vi "WriteScript.vi"() -> ()   [LabVIEW 2015]
panel:
  in  "text file":refnum<file>
  in  "Script Name":string
  out "status":string
  in  "Add to Script Button":bool
  in  "Location of Script File":path
  in  "cluster":T1={"Path to Configuration File"=path "", "SI camera info"={"Exp time"=0.0, "Number of Exp"=0.0, "Exp type tab"=enum."Object", "CCD ROI Mode"=10, "File name base"="", "Camera Color"="Red", "Notes"="", "Observer Name"="", "object name"="", "CCD Readout Speed"=5, "Hg(Ar)"=FALSE, "Cu"=FALSE, "Ne"=FALSE, "Ar"=FALSE, "Quartz"=FALSE, "Fe"=FALSE, "Bulb"=FALSE}} {"SI camera info"."CCD Readout Speed" items=["750 kHz, ATTN 0", "750 kHz, ATTN 2", "344 kHz, ATTN 0", "344 kHz, ATTN 3", "100 kHz, ATTN 2", "100 kHz, ATTN 3"]; "SI camera info"."CCD ROI Mode" items=["Imaging, 1x1  "=0, "Imaging, 2x2"=1, "Imaging, 3x3"=2, "Spectroscopic, 1x1"=3, "Spectroscopic, 2x2"=4, "Spectroscopic, 3x3"=5, "MOS, 1x1"=11, "MOS, 2x2"=12, "MOS, 3x3"=13, "Slicer"=6, "Spectroscopic, ZZ Ceti"=14, "Slit Imaging/Alignment"=7, "MOS Imaging/Alignment"=10, "Set user-defined ROI..."=8, "Custom Mode"=9]}
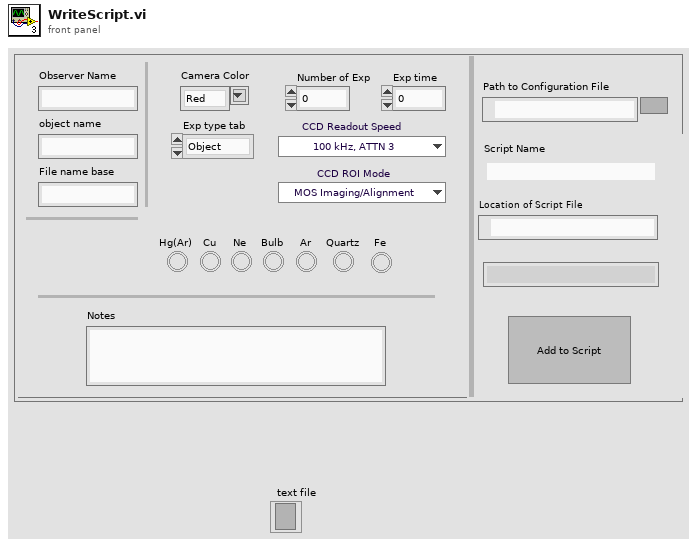
[diagram p1: front panel]
types:
  T1 = cluster{"Path to Configuration File":path, "SI camera info":cluster{"Exp time":dbl, "Number of Exp":dbl, "Exp type tab":enum16{"Object", "Flat", "Comp", "Dark", "Zero"}, "CCD ROI Mode":u16, "File name base":string, "Camera Color":string, "Notes":string, "Observer Name":string, "object name":string, "CCD Readout Speed":u8, "Hg(Ar)":bool, "Cu":bool, "Ne":bool, "Ar":bool, "Quartz":bool, "Fe":bool, "Bulb":bool}}
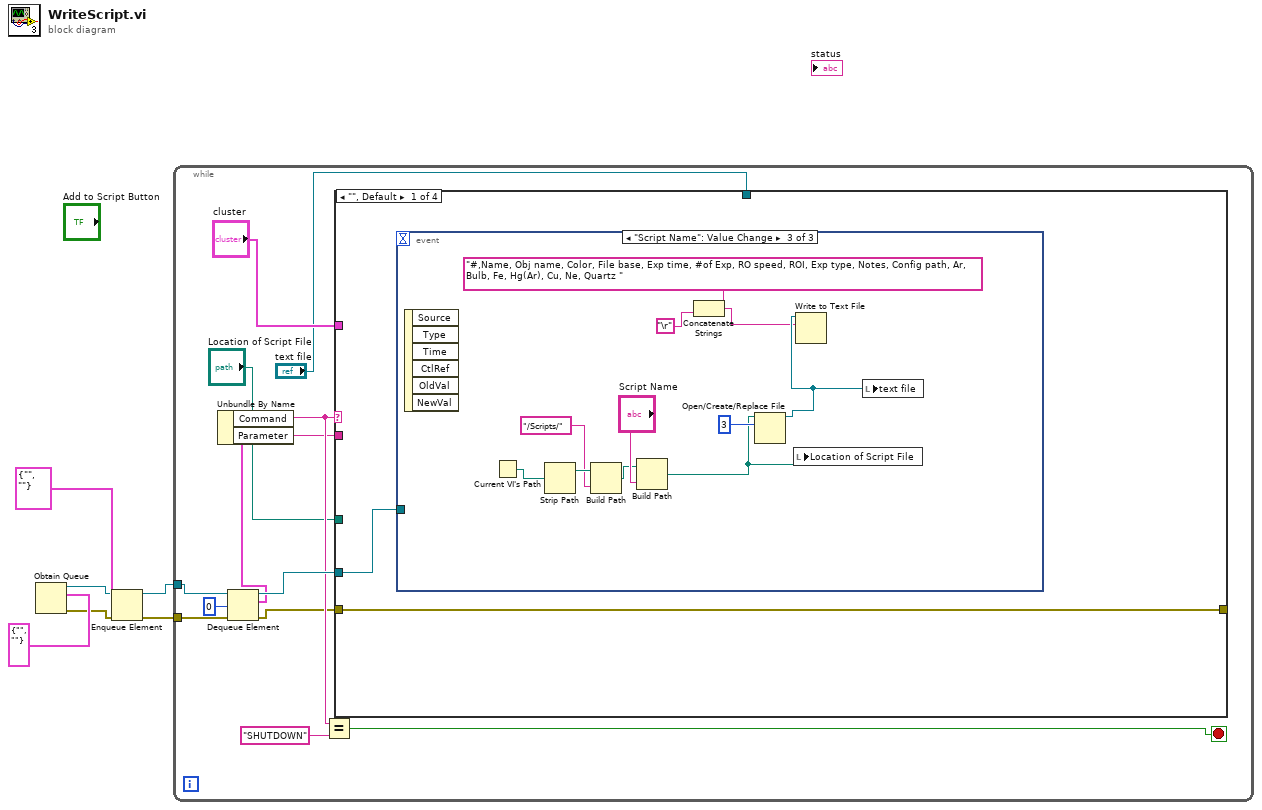
[diagram p0: block diagram]
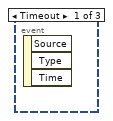
[diagram p2: hidden frame]
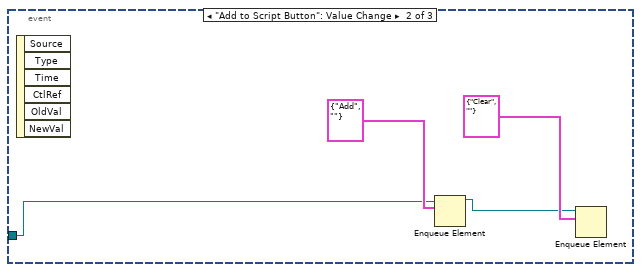
[diagram p3: hidden frame]
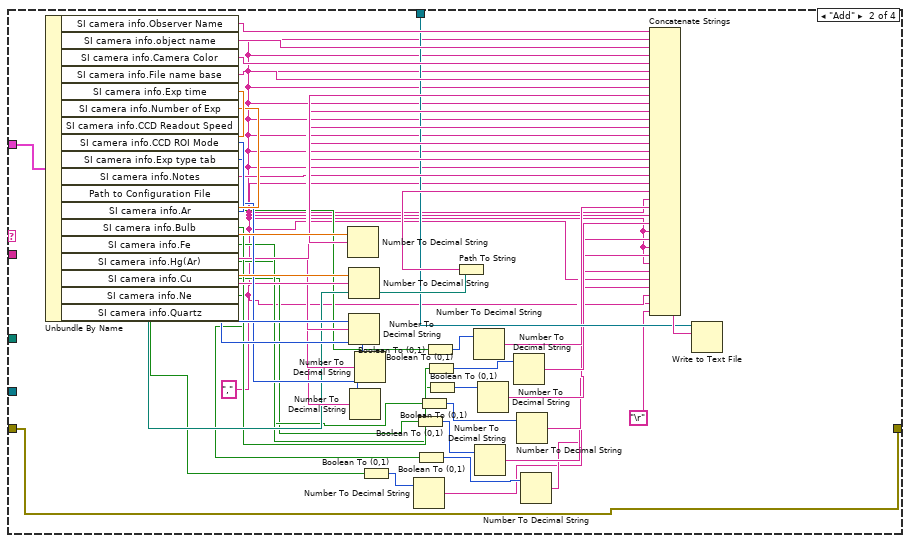
[diagram p4: hidden frame]
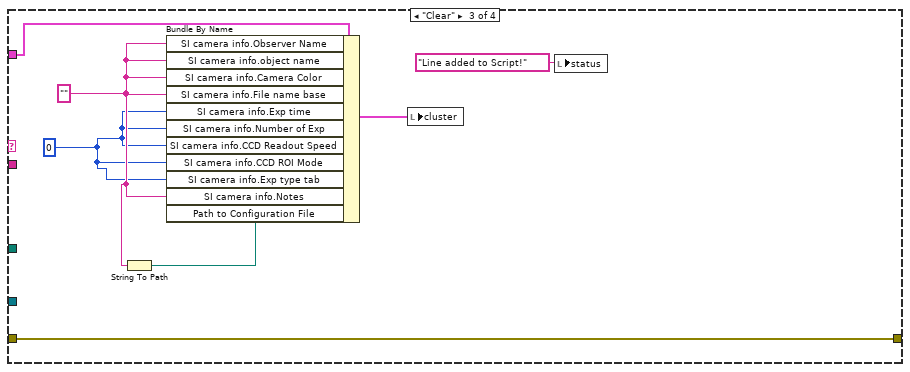
[diagram p5: hidden frame]
diagram:
  n1 = Obtain Queue(element data type=cluster{"\nCommand":string, "Parameter":string} {"\nCommand"="", "Parameter"=""}) -> (queue out=w4:refnum<queue>, error out=w2:errorcluster)  [unwired: 4 in, 1 out]
  n2 = Enqueue Element(queue=w4, element=cluster{string, string} {"", ""}, error in (no error)=w2) -> (queue out=w3:refnum<queue>, error out=w1:errorcluster)  [unwired: 1 in, 1 out]
  n3 = while {
    tunnel: w3 -> [w11]
    tunnel: w1 -> [w10]
    stop <- w15 stop-if-true
    n4 = Dequeue Element(queue=w11, timeout in ms (-1)=0, error in (no error)=w10) -> (queue out=w19:refnum<queue>, element=w18:cluster{"\nCommand":string, "Parameter":string}, error out=w9:errorcluster)  [unwired: 1 out]
    n5 = Unbundle By Name(w18) -> ("Command"=w16:string, "Parameter"=w14:string)
    n6 = Equal?(x=w16, y="SHUTDOWN") -> (x = y?=w15:bool)
    n7 = case shown="\"\", Default" w16 {
      tunnel: w19 -> [w21 _ _ _]
      tunnel: w14 -> [_ _ _ _]
      tunnel: "cluster" -> [_ w80 w87 _]
      tunnel: "Location of Script File" -> [_ _ _ _]
      tunnel: w9 -> [w20 w61 w83 w88]
      tunnel: [w20 w61 w83 w88] -> _
      tunnel: "text file" -> [_ w60 _ _]
      frame "", Default {
        n8 = event shown="[2] \"Script Name\": Value Change" {
          selector: _ -> [_ _ _]
          dyn-events: _ -> [_ _ _]
          timeout: _ -> [_ _ _]
          tunnel: w21 -> [_ w24 _]
          event Timeout {
            n9 = event-data() -> ()  [unwired: 1 in, 3 out]
          }
          event "Add to Script Button": Value Change {
            n10 = event-data() -> ()  [unwired: 1 in, 6 out]
            n11 = Enqueue Element(queue=w24, element=cluster{string, string} {"Add", ""}) -> (queue out=w22:refnum<queue>)  [unwired: 2 in, 2 out]
            n12 = Enqueue Element(queue=w22, element=cluster{string, string} {"Clear", ""}) -> ()  [unwired: 2 in, 3 out]
          }
          event "Script Name": Value Change {
            n13 = event-data() -> ()  [unwired: 1 in, 6 out]
            n14 = Current VI's Path() -> (path=w35:path)
            n15 = Strip Path(path=w35) -> (stripped path=w28:path)  [unwired: 1 out]
            n16 = Build Path(base path=w28, name or relative path="/Scripts/") -> (appended path=w27:path)
            n17 = Build Path(base path=w27, name or relative path="Script Name") -> (appended path=w33:path)
            n18 = Concatenate Strings("#,Name, Obj name, Color, File base, Exp time, #of Exp, RO speed, ROI, Exp type, Notes, Config path, Ar, Bulb, Fe, Hg(Ar), Cu, Ne, Quartz ", "\r") -> (w31:string)
            n19 = Open/Create/Replace File(file path (use dialog)=w33, operation (0:open)=3) -> (refnum out=w32:refnum<file>)  [unwired: 4 in, 2 out]
            n20 = local write "Location of Script File"(w33) -> ()
            n21 = Write to Text File(file (use dialog)=w32, text=w31) -> ()  [unwired: 2 in, 3 out]
            n22 = local write "text file"(w32) -> ()
          }
        }
      }
      frame "Add" {
        w39 = ","
        n23 = Unbundle By Name(w80) -> ("SI camera info.Observer Name"=w79:string, "SI camera info.object name"=w78:string, "SI camera info.Camera Color"=w77:string, "SI camera info.File name base"=w76:string, "SI camera info.Exp time"=w75:dbl, "SI camera info.Number of Exp"=w73:dbl, "SI camera info.CCD Readout Speed"=w72:u8, "SI camera info.CCD ROI Mode"=w71:u16, "SI camera info.Exp type tab"=w70:enum16{"Object", "Flat", "Comp", "Dark", "Zero"}, "SI camera info.Notes"=w65:string, "Path to Configuration File"=w63:path, "SI camera info.Ar"=w59:bool, "SI camera info.Bulb"=w57:bool, "SI camera info.Fe"=w55:bool, "SI camera info.Hg(Ar)"=w53:bool, "SI camera info.Cu"=w51:bool, "SI camera info.Ne"=w49:bool, "SI camera info.Quartz"=w47:bool)
        n24 = Number To Decimal String(number=w75) -> (decimal integer string=w74:string)  [unwired: 1 in]
        n25 = Number To Decimal String(number=w73) -> (decimal integer string=w69:string)  [unwired: 1 in]
        n26 = Number To Decimal String(number=w72) -> (decimal integer string=w68:string)  [unwired: 1 in]
        n27 = Number To Decimal String(number=w70) -> (decimal integer string=w66:string)  [unwired: 1 in]
        n28 = Number To Decimal String(number=w71) -> (decimal integer string=w67:string)  [unwired: 1 in]
        n29 = Boolean To (0,1)(Boolean=w47) -> (0, 1=w46:i16)
        n30 = Number To Decimal String(number=w46) -> (decimal integer string=w38:string)  [unwired: 1 in]
        n31 = Boolean To (0,1)(Boolean=w51) -> (0, 1=w50:i16)
        n32 = Boolean To (0,1)(Boolean=w49) -> (0, 1=w48:i16)
        n33 = Boolean To (0,1)(Boolean=w53) -> (0, 1=w52:i16)
        n34 = Boolean To (0,1)(Boolean=w59) -> (0, 1=w58:i16)
        n35 = Boolean To (0,1)(Boolean=w57) -> (0, 1=w56:i16)
        n36 = Boolean To (0,1)(Boolean=w55) -> (0, 1=w54:i16)
        n37 = Path To String(path=w63) -> (string=w64:string)
        n38 = Number To Decimal String(number=w58) -> (decimal integer string=w45:string)  [unwired: 1 in]
        n39 = Number To Decimal String(number=w50) -> (decimal integer string=w41:string)  [unwired: 1 in]
        n40 = Number To Decimal String(number=w54) -> (decimal integer string=w43:string)  [unwired: 1 in]
        n41 = Number To Decimal String(number=w56) -> (decimal integer string=w44:string)  [unwired: 1 in]
        n42 = Number To Decimal String(number=w52) -> (decimal integer string=w42:string)  [unwired: 1 in]
        n43 = Number To Decimal String(number=w48) -> (decimal integer string=w40:string)  [unwired: 1 in]
        n44 = Concatenate Strings(w79, w39, w78, w39, w77, w39, w76, w39, w74, w39, w69, w39, w68, w39, w67, w39, w66, w39, w65, w39, w64, w39, w45, w39, w44, w39, w43, w39, w42, w39, w41, w39, w40, w39, w38, "\r") -> (w62:string)
        n45 = Write to Text File(file (use dialog)=w60, text=w62) -> ()  [unwired: 2 in, 3 out]
      }
      frame "Clear" {
        w81 = 0
        w84 = ""
        n46 = String To Path(string=w84) -> (path=w85:path)
        n47 = Bundle By Name(cluster=w87, "SI camera info.Observer Name"=w84, "SI camera info.object name"=w84, "SI camera info.Camera Color"=w84, "SI camera info.File name base"=w84, "SI camera info.Exp time"=w81, "SI camera info.Number of Exp"=w81, "SI camera info.CCD Readout Speed"=w81, "SI camera info.CCD ROI Mode"=w81, "SI camera info.Exp type tab"=w81, "SI camera info.Notes"=w84, "Path to Configuration File"=w85) -> (w86:T1)
        n48 = local write "cluster"(w86) -> ()
        n49 = local write "status"("Line added to Script!") -> ()
      }
      frame "Init" {
      }
    }
  }
